vi "roboRIO v1.0 Get Analog Scaling Constants.vi"(8 "error in (no error)":errorcluster, 11 "Analog Channel Name":string) -> (0 "error out":errorcluster, 3 "Analog Scaling Constants":T1)   [LabVIEW 2021]
uses:
  <vilib>/myRIO/Common/Instrument Driver Framework/Utilities/typedefs/Analog Scaling Constants.ctl
  <vilib>/myRIO/Common/Instrument Driver Framework/Utilities/vis/Parse Scaling Constant Table.vi
  <vilib>/myRIO/Common/Instrument Driver Framework/roboRIO v1.0/Resource Manager/vis/roboRIO v1.0 Scaling Constants Table.vi
  <vilib>/Utility/error.llb/Trim Whitespace.vi
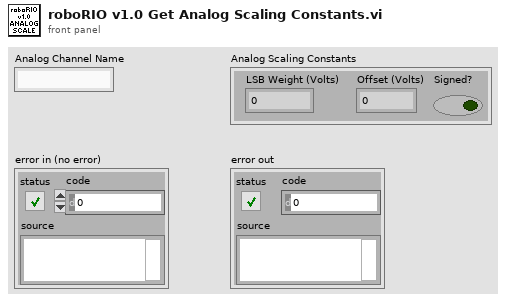
[diagram p1: front panel]
types:
  T1 = typedef "Analog Scaling Constants.ctl" = cluster{"LSB Weight (Volts)":dbl, "Offset (Volts)":dbl, "Signed?":bool}
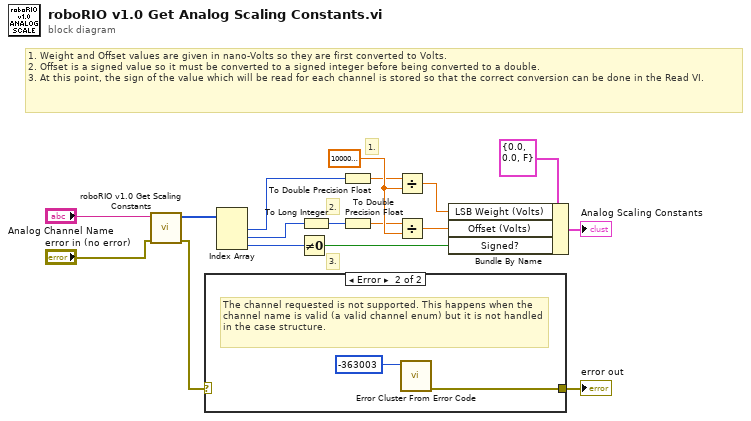
[diagram p0: block diagram]
diagram:
  w10 = 1000000000.0
  # "1. Weight and Offset values are given in nano-Volts so they are first converted to Volts.\n2. Offset is a signed value so it must be converted to a signed integer before being converted to a double.\n3. At this point, the sign of the value which will be read for each channel is stored so that the correct conversion can be done in the Read VI."
  # "3."
  # "2."
  # "1."
  n1 = call <vilib>:"roboRIO v1.0 Get Scaling Constants.vi"("error in (no error)"="error in (no error)", "Channel Name"="Analog Channel Name") -> ("error out"=w2:errorcluster, "Channel Scaling"=w14:u32[])  [unwired: 8 in]
  n2 = case shown="Error" w2 {
    selector: w2 -> [w18 _]
    tunnel: [w18 w19] -> w1
    frame No Error {
    }
    frame Error {
      # "The channel requested is not supported. This happens when the channel name is valid (a valid channel enum) but it is not handled in the case structure."
      n3 = call <vilib>:"Error Cluster From Error Code.vi"("error code (0)"=-363003) -> ("error out"=w19:errorcluster)  [unwired: 8 in]
    }
  }
  "error out" <- w1
  n4 = Index Array(array=w14) -> (element #1=w6:u32, element #2=w5:u32, element #3=w4:u32)  [unwired: 3 in]
  n5 = Not Equal To 0?(x=w4) -> (x != 0?=w3:bool)
  n6 = To Long Integer(number=w5) -> (32bit integer=w7:i32)
  n7 = To Double Precision Float(number=w6) -> (double precision float=w8:dbl)
  n8 = To Double Precision Float(number=w7) -> (double precision float=w9:dbl)
  n9 = Divide(x=w8, y=w10) -> (x/y=w12:dbl)
  n10 = Divide(x=w9, y=w10) -> (x/y=w11:dbl)
  n11 = Bundle By Name(cluster=T1 {"LSB Weight (Volts)"=0.0, "Offset (Volts)"=0.0, "Signed?"=FALSE} ("AI Channel Scaling Constants"), "LSB Weight (Volts)"=w12, "Offset (Volts)"=w11, "Signed?"=w3) -> (→"Analog Scaling Constants":T1)
